vi "SpawnComponentActor.vi"(6 "Unified Actor Alias":string, 7 "Actor in":refnum<class "Actor.lvclass">, 9 "Actors":refnum<class "Actor.lvclass">[](array[class])) -> (0 "Error out":errorcluster, 5 "Actor out":refnum<class "Actor.lvclass">)   [LabVIEW 2020, in "jettl.lvlib"]
uses:
  jettl.lvlib
  Message/Message.lvclass
  Actor.ctl
  ActorLifetime.ctl
  MessageSet.ctl
  ActorRelation.ctl
  MessageMetadata.ctl
  Message.ctl
  Messages.ctl
  Actor/Actor.lvclass
  ActorType.ctl
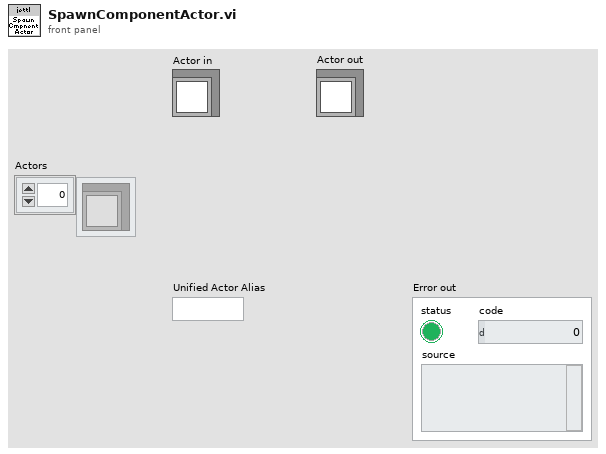
[diagram p1: front panel]
types:
  T1 = typedef "jettl.lvlib/Messages.ctl" = cluster{"Listen":T2, "Tell":T2, "TellSelf":T2, "TellActor":T2}
  T2 = typedef "jettl.lvlib/MessageSet.ctl" = set{refnum<class "Message.lvclass">}
  T3 = typedef "jettl.lvlib/Actor.ctl" = cluster{"Messages":T1, "Alias":string, "Transport":refnum<user-event>, "Address":refnum<event-registration>, "VIRef":refnum<vi>, "ActorType":T4}
  T4 = typedef "jettl.lvlib/ActorType.ctl" = enum16{"Mediator", "Component"}
  T5 = typedef "jettl.lvlib/ActorLifetime.ctl" = enum16{"Init", "Spawn", "Setup", "Teardown Before Running", "Running", "Stop Called", "Stopping With Children", "Stopping Without Children", "Teardown After Running", "Stopped"}
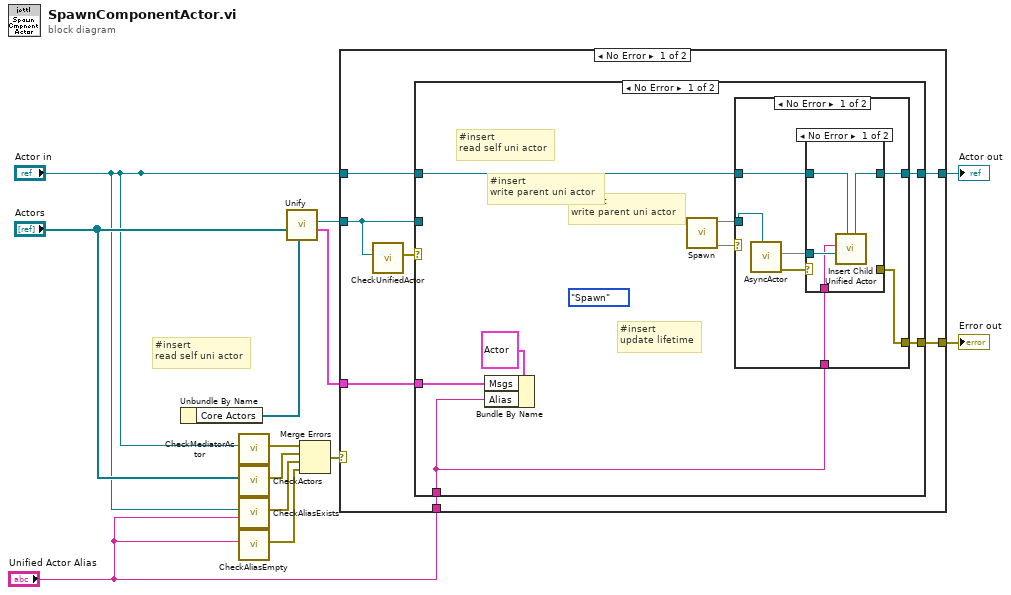
[diagram p0: block diagram]
diagram:
  # "#insert\nread self uni actor"
  n1 = Unbundle By Name() -> ("Core Actors"=w1:refnum<class "Actor.lvclass">[])  [unwired: 1 in]
  n2 = call "CheckMediatorActor.vi"("Actor"="Actor in") -> ("Error"=w13:errorcluster)  [unwired: 10 in]
  n3 = call "CheckActors.vi"("Actors"="Actors") -> ("Error"=w8:errorcluster)  [unwired: 10 in]
  n4 = call "CheckAliasExists.vi"("Alias"="Unified Actor Alias", "Actor"="Actor in") -> ("Error"=w11:errorcluster)  [unwired: 9 in]
  n5 = call "CheckAliasEmpty.vi"("Alias"="Unified Actor Alias") -> ("Error"=w10:errorcluster)  [unwired: 10 in]
  n6 = call "Unify.vi"("Core Actors"=w1, "Mid Actors"="Actors") -> ("Msgs"=w7:T1, "Unified Actor"=w6:refnum<class "Actor.lvclass">)  [unwired: 7 in, 1 out]
  n7 = Merge Errors(w13, w8, w11, w10) -> (w12:errorcluster)
  n8 = case shown="No Error" w12 {
    selector: w12 -> [_ w50]
    tunnel: "Actor in" -> [w16 w51]
    tunnel: [w20 w50] -> w3
    tunnel: [w19 w51] -> w4
    tunnel: "Unified Actor Alias" -> [w18 _]
    tunnel: w7 -> [w15 _]
    tunnel: w6 -> [w14 _]
    frame No Error {
      n9 = call "CheckUnifiedActor.vi"("Unified Actor"=w14) -> ("Error"=w17:errorcluster)  [unwired: 10 in]
      n10 = case shown="No Error" w17 {
        selector: w17 -> [_ w48]
        tunnel: [w32 w48] -> w20
        tunnel: [w31 w49] -> w19
        tunnel: w16 -> [w28 w49]
        tunnel: w18 -> [w27 _]
        tunnel: w15 -> [w29 _]
        tunnel: w14 -> [w23 _]
        frame No Error {
          w22 = ActorLifetime."Spawn" ("Lifetime")
          # "#insert\nupdate lifetime"
          # "#insert\nwrite parent uni actor"
          # "#insert\nread self uni actor"
          # "#insert\nwrite parent uni actor"
          n11 = Bundle By Name(cluster=T3 {"Messages"={"Listen"={}, "Tell"={}, "TellSelf"={}, "TellActor"={}}, "Alias"="", "Transport"=refnum, "Address"=refnum, "VIRef"=refnum, "ActorType"=enum."Mediator"} ("Attributes"), "Msgs"=w29, "Alias"=w27) -> (w26:T3)
          n12 = call-dynamic "Spawn.vi"() -> (0:w24, 3:w25, 11:w21)  [unwired: 7 in, 2 out]
          n13 = case shown="No Error" w24 {
            selector: w24 -> [_ w46]
            tunnel: [w39 w46] -> w32
            tunnel: [w38 w47] -> w31
            tunnel: w28 -> [w37 w47]
            tunnel: w25 -> [w35 _]
            tunnel: w27 -> [w33 _]
            frame No Error {
              n14 = call "AsyncActor.vi"("Actor in"=w35) -> ("Error out"=w36:errorcluster, 2:w34)  [unwired: 9 in]
              n15 = case shown="No Error" w36 {
                selector: w36 -> [_ w44]
                tunnel: w37 -> [w43 w45]
                tunnel: [w42 w45] -> w38
                tunnel: w34 -> [w41 _]
                tunnel: [_ w44] -> w39
                tunnel: w33 -> [w40 _]
                frame No Error {
                  n16 = call "Insert Child Unified Actor.vi"("Actor in"=w43, "Child Unified Actor"=w41, "Unified Actor Alias"=w40) -> ("Actor out"=w42:refnum<class "Actor.lvclass">)  [unwired: 8 in]
                }
                frame Error {
                }
              }
            }
            frame Error {
            }
          }
        }
        frame Error {
        }
      }
    }
    frame Error {
    }
  }
  "Actor out" <- w4
  "Error out" <- w3
